vi "notifyTaskState.vi"(7 "TaskName":string, 8 "error in (no error)":errorcluster, 9 "Data":variant, 10 "Request":string, 11 "pdbm_testsystem_feeback_event":refnum<user-event>) -> (0 "error out":errorcluster, 3 "pdbm_testsystem_feeback_event out":refnum<user-event>)   [LabVIEW 2015, in "pdbm_test_system.lvlib"]
uses:
  pdbm_test_system.lvlib
  UsrDefine/pdbm_testsystem_feedback_data.ctl
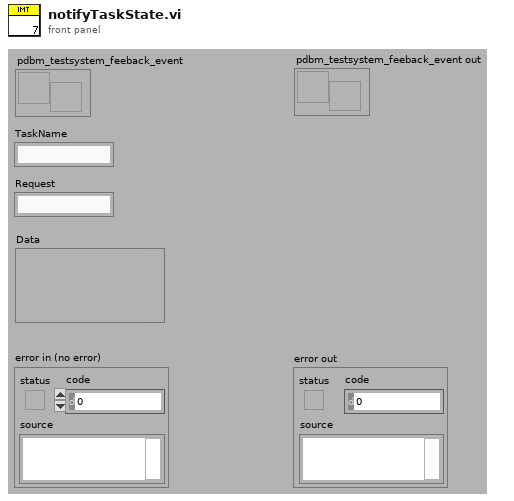
[diagram p1: front panel]
types:
  T1 = typedef "pdbm_test_system.lvlib/pdbm_testsystem_feedback_data.ctl" = cluster{"TaskName":string, "Request":string, "Data":variant}
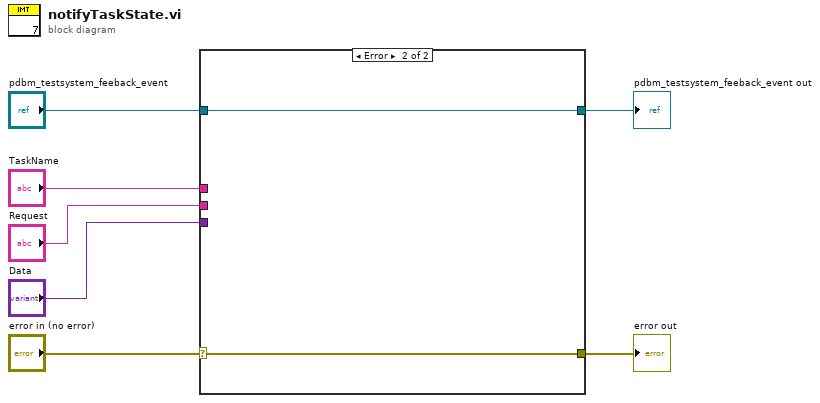
[diagram p0: block diagram]
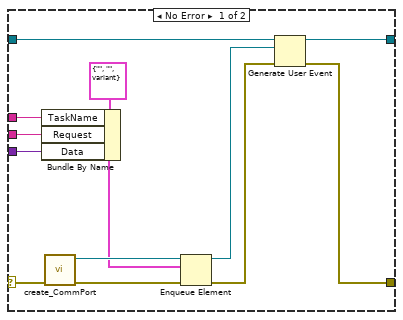
[diagram p2: hidden frame]
diagram:
  n1 = case shown="Error" "error in (no error)" {
    selector: "error in (no error)" -> [w8 w21]
    tunnel: "TaskName" -> [w19 _]
    tunnel: "Request" -> [w18 _]
    tunnel: "Data" -> [w17 _]
    tunnel: "pdbm_testsystem_feeback_event" -> [w13 w22]
    tunnel: [w10 w22] -> w3
    tunnel: [w9 w21] -> w2
    frame No Error {
      n2 = Bundle By Name(cluster=T1 {"TaskName"="", "Request"="", "Data"=variant} ("pdbm_test_system_feedback data"), "TaskName"=w19, "Request"=w18, "Data"=w17) -> (w14:T1)
      n3 = call "create_CommPort.vi"("error in (no error)"=w8) -> ("error out"=w15:errorcluster, "pdbm_testsys_feedback_event"=w16:refnum<queue>)  [unwired: 9 in]
      n4 = Enqueue Element(queue=w16, element=w14, error in (no error)=w15) -> (queue out=w12:refnum<queue>, error out=w11:errorcluster)  [unwired: 1 in, 1 out]
      n5 = Generate User Event(user event=w13, event data cluster=w12, error in=w11) -> (user event out=w10:refnum<user-event>, error out=w9:errorcluster)  [unwired: 1 in]
    }
    frame Error {
    }
  }
  "pdbm_testsystem_feeback_event out" <- w3
  "error out" <- w2
